vi "Read FPGA_Ref.vi"(8 "error in":errorcluster, 11 "Combined PAS in":refnum<class "cPAS.lvclass">) -> (0 "error out":errorcluster, 2 "FPGA VI Reference Out":T1, 3 "Combined PAS out":refnum<class "cPAS.lvclass">)   [LabVIEW 2015, in "cPAS.lvclass"]
uses:
  cPAS.lvclass
  Interface/fpga_ctl.ctl
  cPAS.lvclass/cPAS.ctl
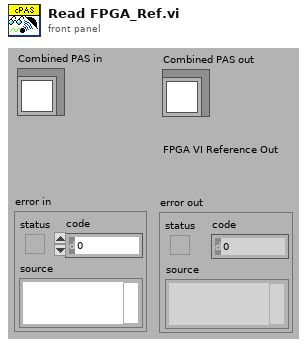
[diagram p1: front panel]
types:
  T1 = typedef "fpga_ctl.ctl" = refnum<k20>
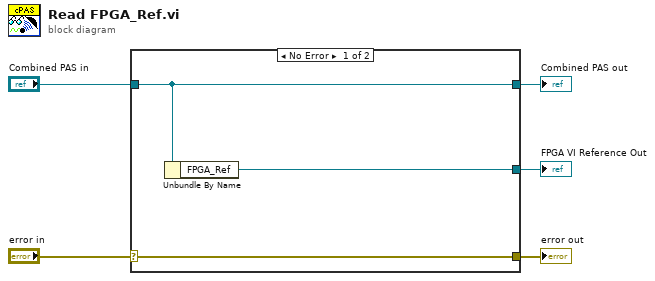
[diagram p0: block diagram]
diagram:
  n1 = case shown="No Error" "error in" {
    selector: "error in" -> [w8 w9]
    tunnel: [w8 w9] -> w4
    tunnel: [w7 w10] -> w2
    tunnel: "Combined PAS in" -> [w7 w10]
    tunnel: [w6 _] -> w1
    frame No Error {
      n2 = Unbundle By Name(w7) -> ("FPGA_Ref"=w6:T1)
    }
    frame Error {
    }
  }
  "error out" <- w4
  "Combined PAS out" <- w2
  "FPGA VI Reference Out" <- w1
